vi "WriteDataToDB 1.vi"(8 "通信协议名称":string, 9 "SN":string, 10 "产品型号":string, 11 "Slot":T1) -> (2 "ResultA":string, 3 "FSNA":string)   [LabVIEW 2013]
uses:
  SystemCode/SysControl/Slot.ctl
  GlobalValue.vi
  <vilib>/Utility/file.llb/Write To Spreadsheet File (string).vi
  <vilib>/Utility/file.llb/Read From Spreadsheet File (string).vi
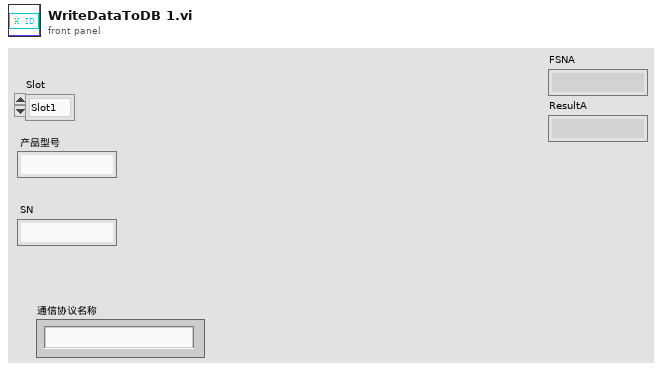
[diagram p1: front panel]
types:
  T1 = typedef "Slot.ctl" = enum16{"Slot1", "Slot2", "Slot3", "Slot4"}
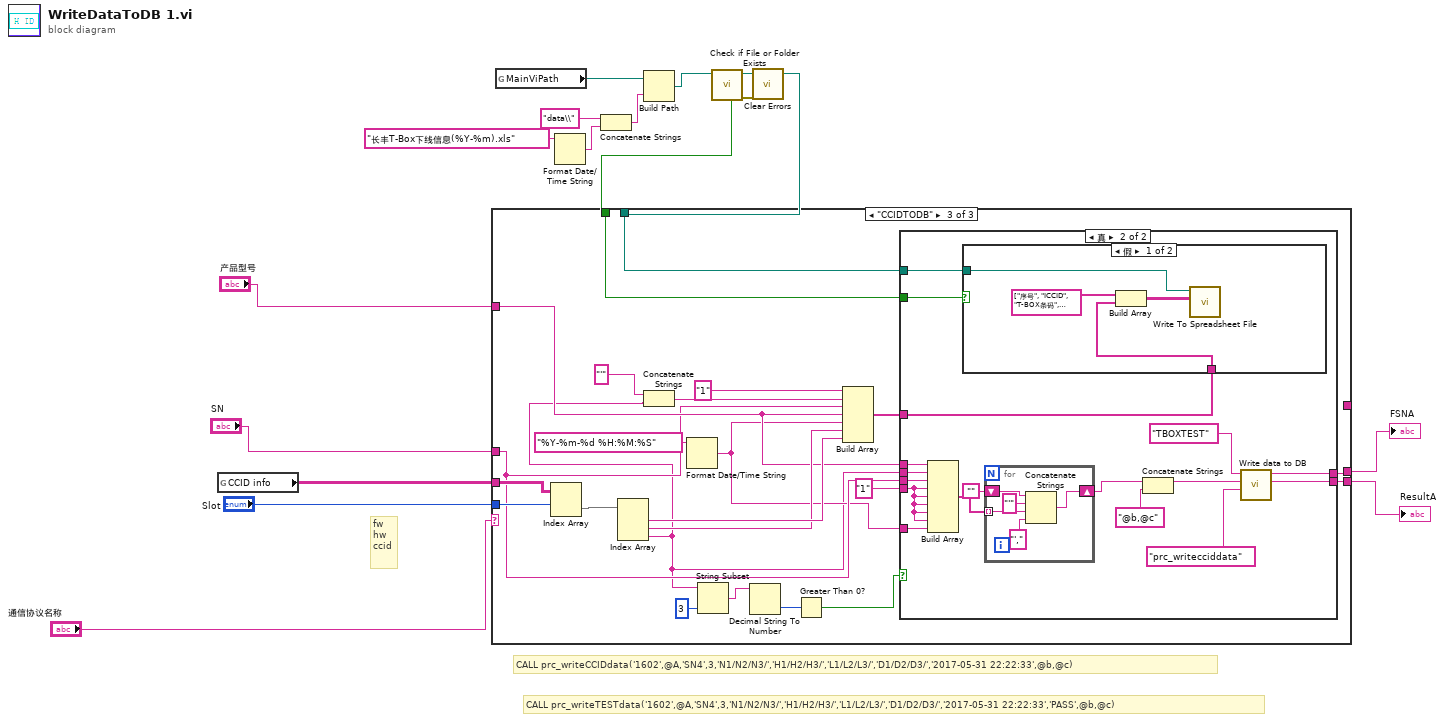
[diagram p0: block diagram]
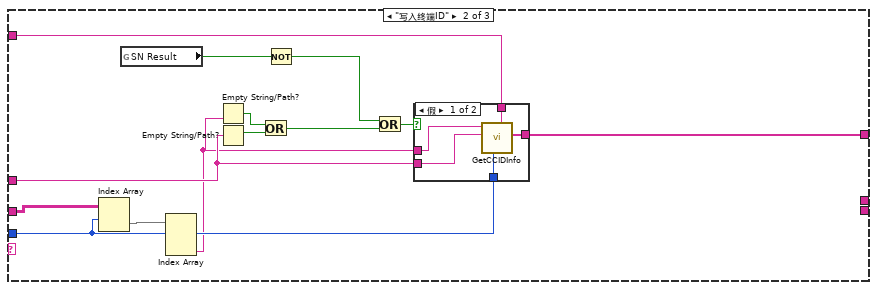
[diagram p3: hidden frame]
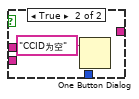
[diagram p4: hidden frame]
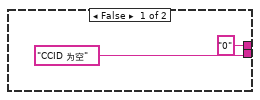
[diagram p5: hidden frame]
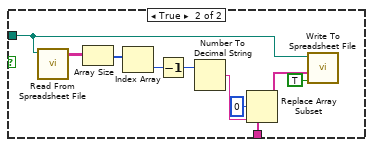
[diagram p6: hidden frame]
diagram:
  # "CALL prc_writeCCIDdata('1602',@A,'SN4',3,'N1/N2/N3/','H1/H2/H3/','L1/L2/L3/','D1/D2/D3/','2017-05-31 22:22:33',@b,@c)"
  # "CALL prc_writeTESTdata('1602',@A,'SN4',3,'N1/N2/N3/','H1/H2/H3/','L1/L2/L3/','D1/D2/D3/','2017-05-31 22:22:33','PASS',@b,@c)"
  # "fw\nhw\nccid"
  n1 = global read "GlobalValue.vi" "CCID info"() -> (w6:string[][])
  n2 = global read "GlobalValue.vi" "MainViPath"() -> (w13:path)
  n3 = Format Date/Time String(time format string (%c)="长丰T-Box下线信息(%Y-%m).xls" ("时间格式字符串(%c)")) -> (date/time string=w15:string)  [unwired: 2 in]
  n4 = Concatenate Strings("data\\" ("字符串"), w15) -> (w12:string)
  n5 = Build Path(base path=w13, name or relative path=w12) -> (appended path=w11:path)
  n6 = call <vilib>:"Check if File or Folder Exists.vi"("path"=w11) -> ("error out"=w10:errorcluster, "file or folder exists?"=w9:bool, "dup path"=w8:path)  [unwired: 8 in]
  n7 = case shown="\"CCIDTODB\"" "通信协议名称" {
    tunnel: [_ w29 _] -> _
    tunnel: "产品型号" -> [_ w22 w46]
    tunnel: w8 -> [_ _ w55]
    tunnel: w9 -> [_ _ w54]
    tunnel: "SN" -> [_ w21 w45]
    tunnel: "Slot" -> [_ w18 w50]
    tunnel: w6 -> [_ w19 w51]
    tunnel: [_ _ w42] -> w4
    tunnel: [_ _ w41] -> w3
    frame "假", Default {
    }
    frame "写入终端ID" {
      n8 = Index Array(array=w19, index (row)=w18) -> (element=w20:string[])  [unwired: 1 in]
      n9 = global read "GlobalValue.vi" "SN Result"() -> (w28:bool)
      n10 = Index Array(array=w20) -> (element #3=w17:string)  [unwired: 3 in, 2 out]
      n11 = Empty String/Path?(string/path=w17) -> (empty?=w27:bool)
      n12 = Empty String/Path?(string/path=w21) -> (empty?=w26:bool)
      n13 = Or(x=w27, y=w26) -> (x .or. y?=w24:bool)
      n14 = Not(x=w28) -> (.not. x?=w25:bool)
      n15 = Or(x=w25, y=w24) -> (x .or. y?=w23:bool)
      n16 = case shown="假" w23 {
        tunnel: [w34 _] -> w29
        tunnel: w17 -> [w33 _]
        tunnel: w21 -> [w32 _]
        tunnel: w22 -> [w31 _]
        tunnel: w18 -> [w30 _]
        frame False {
          n17 = call "GetCCIDInfo.vi"("table name"=w31, "Slot"=w30, "SerNO"=w32, "CCID"=w33) -> ("CCID信息"=w34:string[])  [unwired: 7 in]
        }
        frame True {
          n18 = One Button Dialog(message="CCID为空" ("消息")) -> ()  [unwired: 1 in, 1 out]
        }
      }
    }
    frame "CCIDTODB" {
      n19 = Index Array(array=w51, index (row)=w50) -> (element=w49:string[])  [unwired: 1 in]
      n20 = Index Array(array=w49) -> (element #1=w48:string, element #2=w47:string, element #3=w40:string)  [unwired: 3 in]
      n21 = Concatenate Strings("'", w40) -> (w52:string)
      n22 = Format Date/Time String(time format string (%c)="%Y-%m-%d %H:%M:%S" ("时间格式字符串(%c)")) -> (date/time string=w44:string)  [unwired: 2 in]
      n23 = String Subset(string=w40, length (rest)=3 ("长度（剩余）")) -> (substring=w38:string)  [unwired: 1 in]
      n24 = Decimal String To Number(string=w38) -> (number=w37:i32)  [unwired: 2 in, 1 out]
      n25 = Greater Than 0?(x=w37) -> (x > 0?=w36:bool)
      n26 = Build Array("1", w52, w45, w46, w44, w47, w48) -> (w56:string[])
      n27 = case shown="真" w36 {
        tunnel: w56 -> [_ w77]
        tunnel: w55 -> [_ w76]
        tunnel: w54 -> [_ w75]
        tunnel: w46 -> [_ w72]
        tunnel: w45 -> [_ w71]
        tunnel: w44 -> [_ w70]
        tunnel: "1" ("元素") -> [_ w69]
        tunnel: ["0" ("FSNA") w63] -> w42
        tunnel: ["CCID 为空" ("ResultA") w62] -> w41
        tunnel: w40 -> [_ w61]
        frame False {
        }
        frame True {
          n28 = Build Array(w72, w61, w71, w69, w69, w69, w69, w69, w70) -> (w68:string[])
          n29 = case shown="假" w75 {
            tunnel: w76 -> [w86 w87]
            tunnel: w77 -> [w85 w91]
            frame False {
              n30 = Build Array(string[] ["序号", "ICCID", "T-BOX条码", "设备型号", "生产日期", "硬件版本", "软件版本"], w85) -> (w84:string[][])
              n31 = call-poly <vilib>:"Write To Spreadsheet File.vi"("2D data"=w84, "file path (dialog if empty)"=w86) -> ()  [unwired: 6 in, 1 out]
            }
            frame True {
              n32 = call-poly <vilib>:"Read From Spreadsheet File.vi"("file path (dialog if empty)"=w87) -> ("all rows"=w96:string[][])  [unwired: 6 in, 4 out]
              n33 = Array Size(array=w96) -> (size(s)=w95:i32[])
              n34 = Index Array(array=w95) -> (element=w94:i32)  [unwired: 1 in]
              n35 = Decrement(x=w94) -> (x-1=w93:i32)
              n36 = Number To Decimal String(number=w93) -> (decimal integer string=w89:string)  [unwired: 1 in]
              n37 = Replace Array Subset(array=w91, new element=w89, index=0 ("索引")) -> (w88:string[])
              n38 = call-poly <vilib>:"Write To Spreadsheet File.vi"("append to file? (new file:F)"=TRUE, "1D data"=w88, "file path (dialog if empty)"=w87) -> ()  [unwired: 5 in, 1 out]
            }
          }
          n39 = for {
            tunnel: w68 -> [w79] mode=indexing
            shift-right: [w81] -> w66
            shift-left: "" -> [w80]
            n40 = Concatenate Strings(w80, "'" ("字符串"), w79, "',") -> (w81:string)
          }
          n41 = Concatenate Strings(w66, "@b,@c" ("元素")) -> (w64:string)
          n42 = call "Write data to DB.vi"("Procedure name"="prc_writecciddata", "all string"=w64, "DSN name"="TBOXTEST") -> ("ResultA"=w62:string, "FSNA"=w63:string)  [unwired: 6 in, 1 out]
        }
      }
    }
  }
  "FSNA" <- w4
  "ResultA" <- w3
  n43 = call <vilib>:"Clear Errors.vi"("error in (no error)"=w10) -> ()  [unwired: 6 in, 1 out]
